vi "UAGetClientCerts.vi"(8 "error in (no error)":errorcluster, 11 "trustedClientCertifications data":string) -> (0 "error out":errorcluster, 3 "Array":path[](array[path]))   [LabVIEW 2014, in "OPCUA XML(dev).lvlib"]
uses:
  OPCUA XML(dev).lvlib
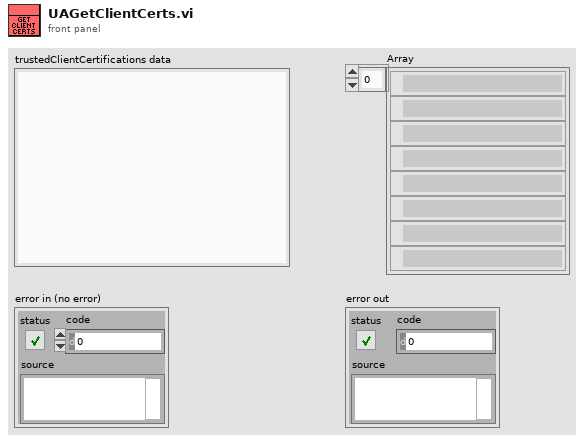
[diagram p1: front panel]
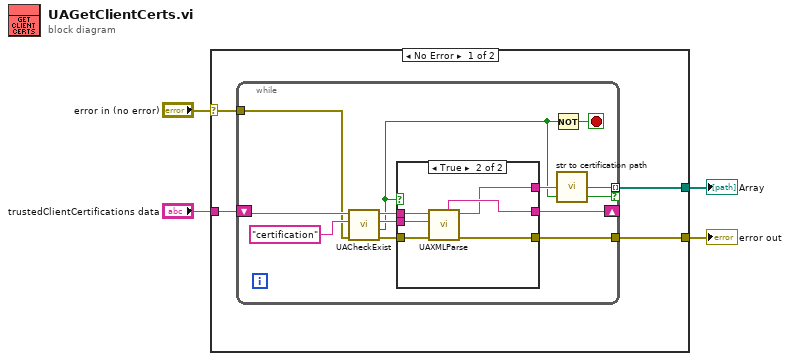
[diagram p0: block diagram]
diagram:
  n1 = case shown="No Error" "error in (no error)" {
    selector: "error in (no error)" -> [w5 w29]
    tunnel: [w8 w29] -> w4
    tunnel: [w7 _] -> w3
    tunnel: "trustedClientCertifications data" -> [w6 _]
    frame No Error {
      n2 = while {
        shift-right: [w20] -> _
        shift-left: w6 -> [w16]
        tunnel: [w13] -> w7 mode=indexing if=w9
        tunnel: w5 -> [w12]
        tunnel: [w11] -> w8
        stop <- w10 stop-if-true
        n3 = call "UACheckExist.vi"("error in (no error)"=w12, "label"="certification", "string"=w16) -> ("error out"=w14:errorcluster, "exist?"=w9:bool, "label (dup)"=w17:string, "string (dup)"=w18:string)  [unwired: 5 in]
        n4 = case shown="True" w9 {
          tunnel: [w22 w28] -> w20
          tunnel: [_ w27] -> w19
          tunnel: w18 -> [w22 w26]
          tunnel: w17 -> [_ w25]
          tunnel: w14 -> [w21 w24]
          tunnel: [w21 w23] -> w11
          frame False {
          }
          frame True {
            n5 = call "UAXMLParse.vi"("error in (no error)"=w24, "label"=w25, "string"=w26) -> ("error out"=w23:errorcluster, "content"=w27:string, "after substring"=w28:string)  [unwired: 3 in, 3 out]
          }
        }
        n6 = Not(x=w9) -> (.not. x?=w10:bool)
        n7 = call "str to certification path.vi"("node text"=w19) -> ("File Path Control"=w13:path)  [unwired: 4 in]
      }
    }
    frame Error {
    }
  }
  "error out" <- w4
  "Array" <- w3
